vi "remove earth field.vi"(10 "earth magnetic field":cluster{"x":dbl, "y":dbl}, 11 "mag data":T1[](array[typedef])) -> (3 "mag data earth field subtracted":T1[](array[typedef]))   [LabVIEW 2017]
uses:
  typedefs/reading3.ctl
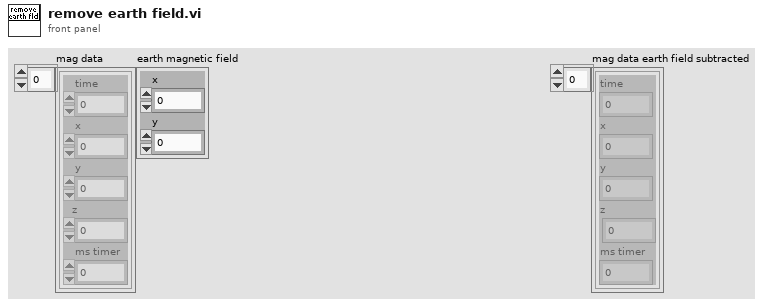
[diagram p1: front panel]
types:
  T1 = typedef "reading3.ctl" = cluster{"time":dbl, "x":dbl, "y":dbl, "z":dbl, "ms timer":u32}
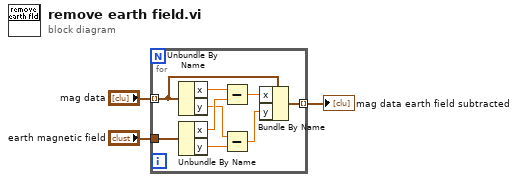
[diagram p0: block diagram]
diagram:
  n1 = for {
    tunnel: "mag data" -> [w7] mode=indexing
    tunnel: "earth magnetic field" -> [w12]
    tunnel: [w4] -> w1 mode=indexing
    n2 = Unbundle By Name(w7) -> ("x"=w11:dbl, "y"=w9:dbl)
    n3 = Unbundle By Name(w12) -> ("x"=w10:dbl, "y"=w8:dbl)
    n4 = Subtract(x=w11, y=w10) -> (x-y=w6:dbl)
    n5 = Subtract(x=w9, y=w8) -> (x-y=w5:dbl)
    n6 = Bundle By Name(cluster=w7, "x"=w6, "y"=w5) -> (w4:T1)
  }
  "mag data earth field subtracted" <- w1
